vi "Get_Robot_And_Goal_Heading(SubVI).vi"(11 "Current_Position":T1) -> (3 "heading":T2)   [LabVIEW 2017]
doc: "Get and bundle robot's current heading and goal heading"
uses:
  Ctl/Current_Position.ctl
  GBL/GBL_variables.vi
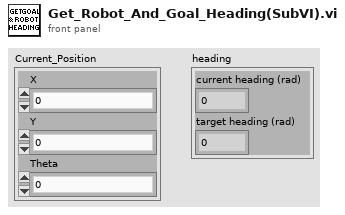
[diagram p1: front panel]
types:
  T1 = typedef "Current_Position.ctl" = cluster{"X":dbl, "Y":dbl, "Theta":dbl}
  T2 = cluster{"current heading (rad)":dbl, "target heading (rad)":dbl}
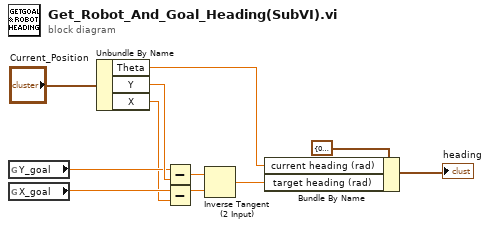
[diagram p0: block diagram]
diagram:
  n1 = global read "GBL_variables.vi" "Y_goal"() -> (w3:dbl)
  n2 = global read "GBL_variables.vi" "X_goal"() -> (w6:dbl)
  n3 = Unbundle By Name("Current_Position") -> ("Theta"=w10:dbl, "Y"=w5:dbl, "X"=w1:dbl)
  n4 = Subtract(x=w3, y=w5) -> (x-y=w4:dbl)
  n5 = Subtract(x=w6, y=w1) -> (x-y=w2:dbl)
  n6 = Inverse Tangent (2 Input)(1:w2, 2:w4) -> (0:w7:dbl)
  n7 = Bundle By Name(cluster=T2 {"current heading (rad)"=0.0, "target heading (rad)"=0.0} ("heading"), "current heading (rad)"=w10, "target heading (rad)"=w7) -> (→"heading":T2)
